vi "Init (Key).vi"(6 "Index (:TODO:)":i32=-1, 8 "error in (no error)":errorcluster, 9 "Value":string, 10 "Name":string) -> (0 "error out":errorcluster, 3 "Find First Query out":refnum<class "Insert Query.lvclass">)   [LabVIEW 2013, in "Insert Query.lvclass"]
doc: "Copyright 2018, Carya Automatisering, Wiebe Walstra."
uses:
  Insert Query.lvclass
  Data.ctl
  Insert Query.lvclass/Insert Query.ctl
  CConfig Object.lvclass
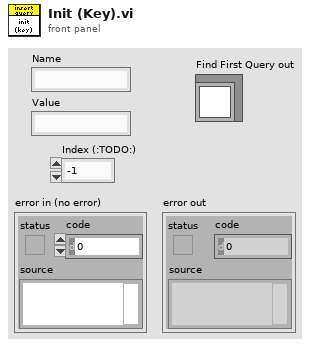
[diagram p1: front panel]
types:
  T1 = typedef "CConfig Object.lvclass/Data.ctl" = enum16{"pre", "name", "middle", "value", "post", "newline", "persistant", "tagged", "type"}
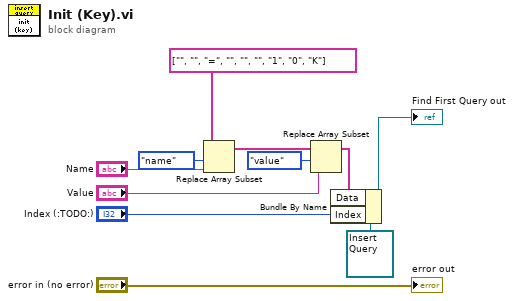
[diagram p0: block diagram]
diagram:
  n1 = Replace Array Subset(array=string[] ["", "", "=", "", "", "", "1", "0", "K"] ("Data"), new element="Name", index=Data."name" ("Data")) -> (w6:string[])
  n2 = Replace Array Subset(array=w6, new element="Value", index=Data."value" ("Data")) -> (w5:string[])
  n3 = Bundle By Name(cluster=refnum<class "Insert Query.lvclass"> refnum ("Find First Query in"), "Data"=w5, "Index"="Index (:TODO:)") -> (→"Find First Query out":refnum<class "Insert Query.lvclass">)
  "error out" <- "error in (no error)"
